vi "Graph_Peak_testing.vi"(6 "CSV file path":path, 7 "error in":errorcluster, 10 "Cluster":T2) -> (0 "MIN_MAX_BPM":bool, 2 "Filter Graph":cluster{timestamp[], ext[]}(graph), 3 "MIN_MAX_PRESSURE":bool, 4 "ACTUAL BPM":dbl, 5 "error out":errorcluster, 8 "MAX_MIN_PRESSURE":cluster{"MIN":dbl, "MAX":dbl, "ACTUAL":dbl}, 9 "UnFiltered \nSize":i32)   [LabVIEW 2017]
uses:
  <vilib>/Utility/file.llb/Read Delimited Spreadsheet (string).vi
panel:
  out "Pressure":T1
  out "ACTUAL":ext
  out "max value 2":ext
  out "max value":ext
  out "Peak samples / second":dbl
  out "time in sec between start peak stop peak":dbl
  out "Array 14":ext[](array[numeric])
  out "Array":timestamp[](array[timestamp])
  out "input filter array":ext[](array[numeric])
  out "Normal Graph":cluster{timestamp[], ext[]}(graph)
  out "Numeric 3":i32
  out "Numeric":i32
  out "Array 13":ext[][](array[numeric])
  out "Array 12":ext[](array[numeric])
  out "appended array 2":timestamp[][](array[timestamp])
  out "peak count":i32
  out "Array 11":ext[](array[numeric])
  out "Array 8":timestamp[](array[timestamp])
  out "appended array":timestamp[][](array[timestamp])
  out "Array 9":ext[][](array[numeric])
  out "Input\nLower\nthan\nthreshold":bool
  out "Filtered \nSize":i32
  out "STOP\nTHRESHOLD\nTRIGGER\nindex":i32
  out "START\nTHRESHOLD\nTRIGGER\nindex":i32
  out "time stamp":timestamp[](array[timestamp])
  out "input unfilter array":ext[](array[numeric])
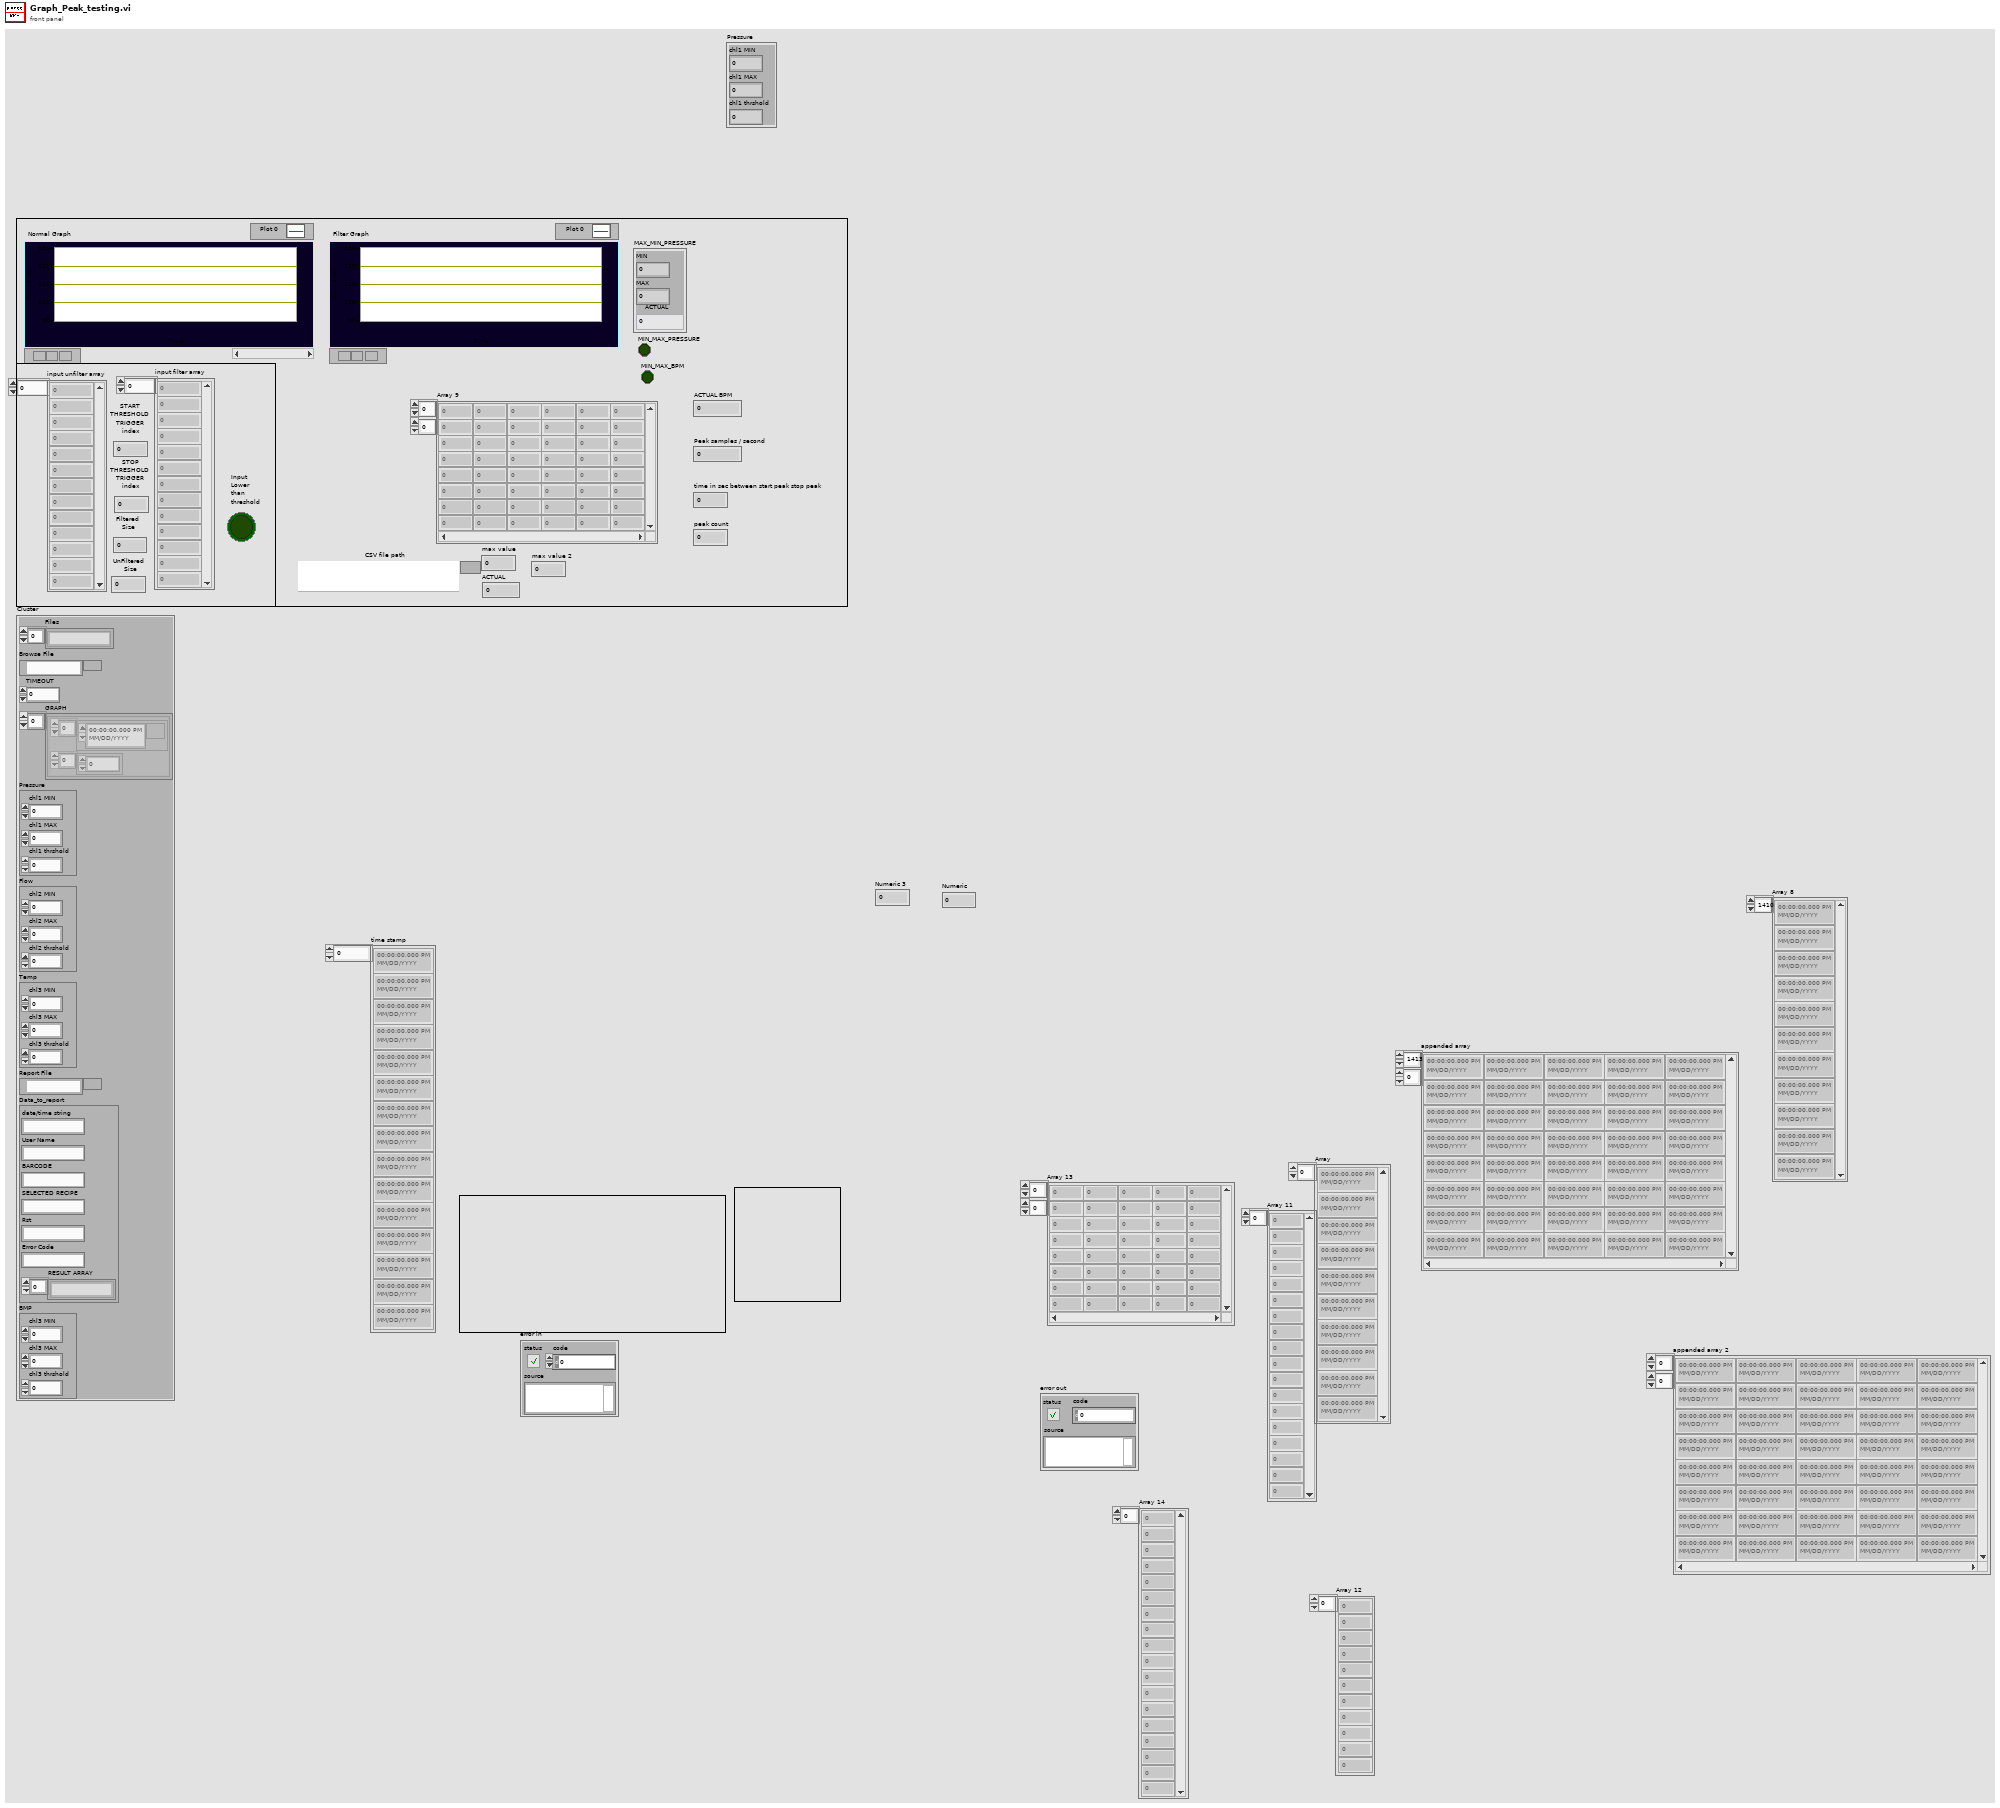
[diagram p1: front panel]
types:
  T1 = cluster{"chl1 MIN":dbl, "chl1 MAX":dbl, "chl1 thrshold":dbl}
  T2 = cluster{"Files":string[], "Browse File":path, "TIMEOUT":i32, "GRAPH":cluster{timestamp[], ext[]}[], "Pressure":cluster{"chl1 MIN":dbl, "chl1 MAX":dbl, "chl1 thrshold":dbl}, "Flow":cluster{"chl2 MIN":dbl, "chl2 MAX":dbl, "chl2 thrshold":dbl}, "Temp":cluster{"chl3 MIN":dbl, "chl3 MAX":dbl, "chl3 thrshold":dbl}, "Report File":path, "Data_to_report":cluster{"date/time string":string, "User Name":string, "BARCODE":string, "SELECTED RECIPE":string, "Rst":string, "Error Code":string, "RESULT ARRAY":string[]}, "BMP":cluster{"chl3 MIN":dbl, "chl3 MAX":dbl, "chl3 thrshold":dbl}}
  T3 = cluster{"chl3 MIN":dbl, "chl3 MAX":dbl, "chl3 thrshold":dbl}
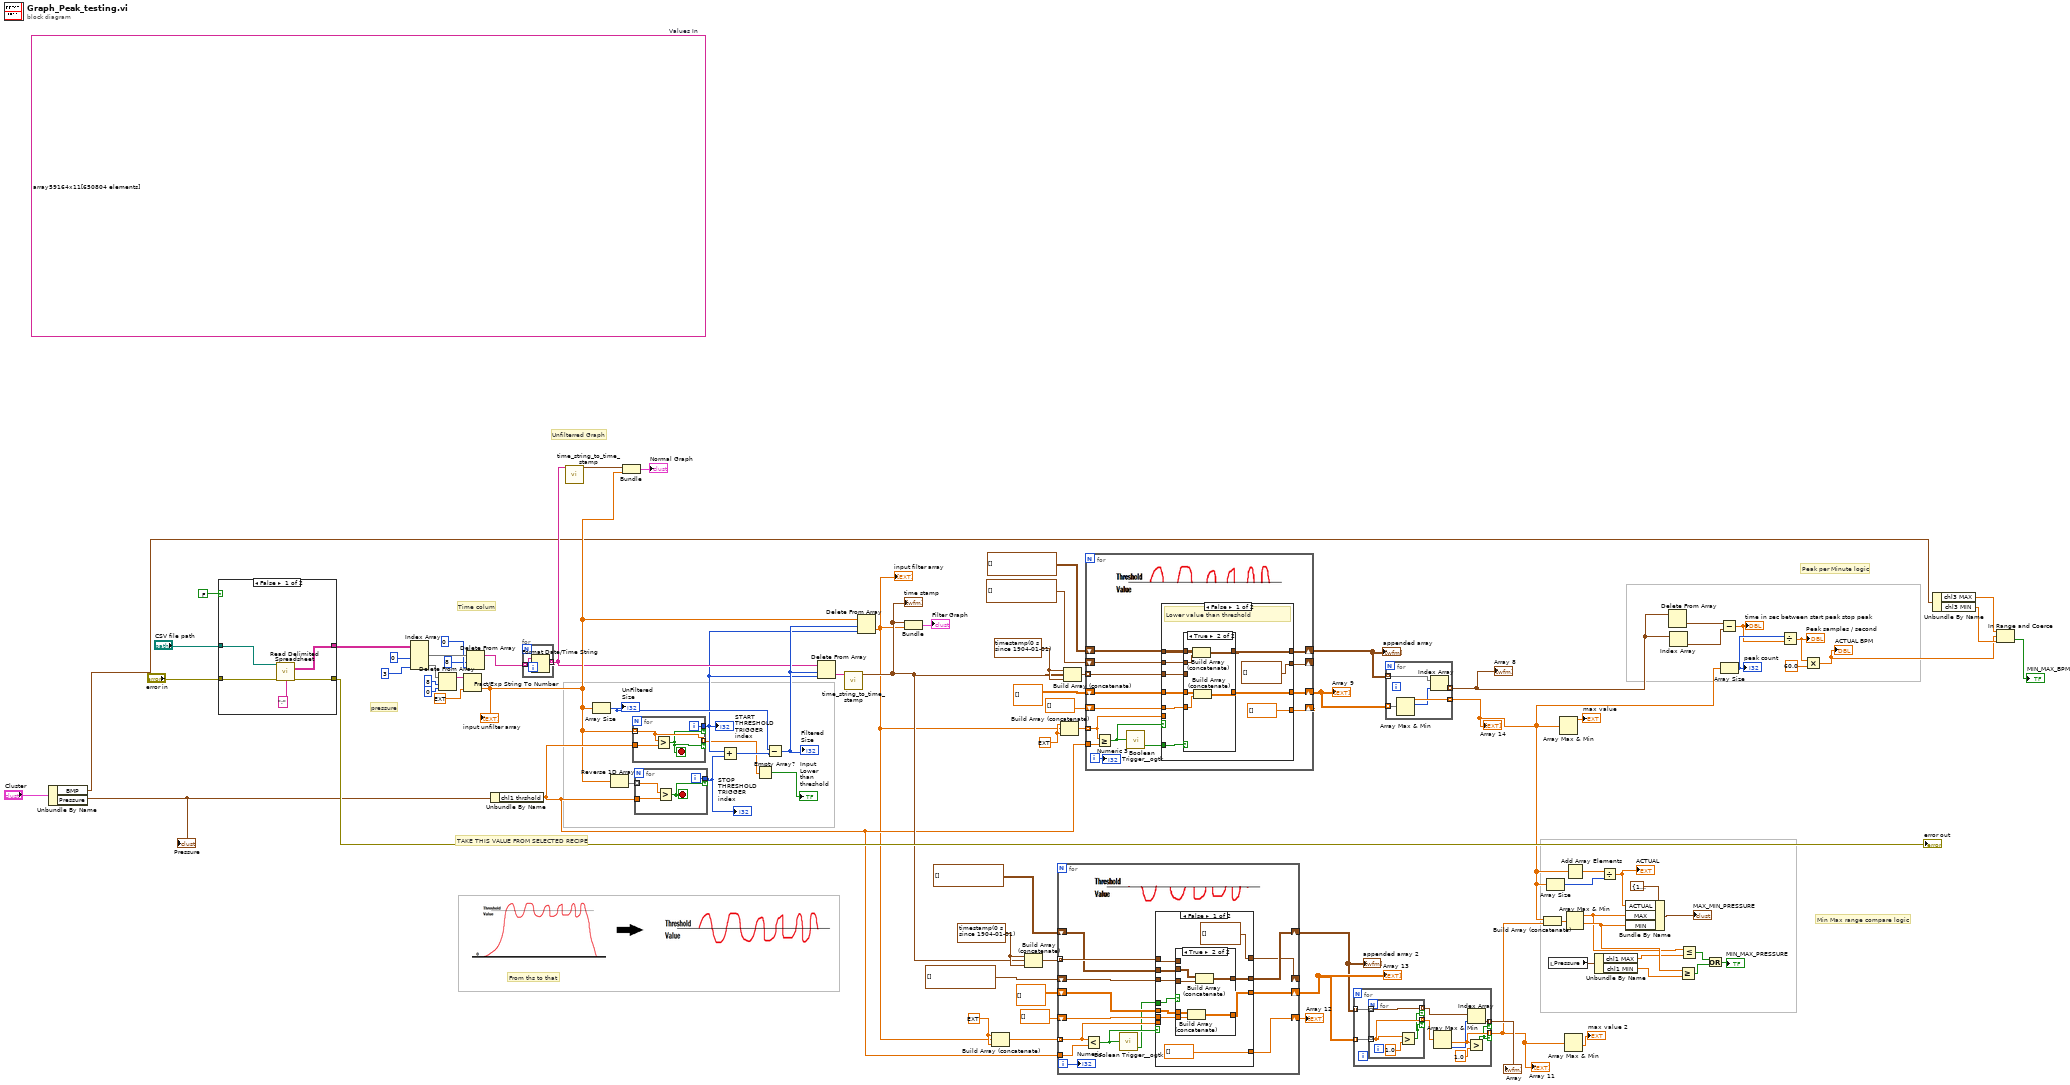
[diagram p0: block diagram]
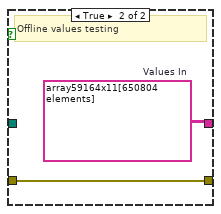
[diagram p2: hidden frame]
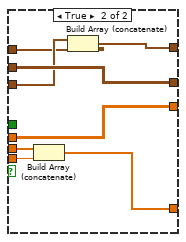
[diagram p4: hidden frame]
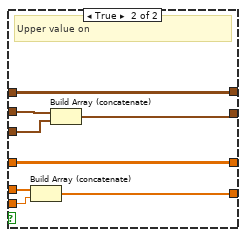
[diagram p6: hidden frame]
diagram:
  (unwired) string[][] array59164x11[650804 elements]  # Values In
  w62 = timestamp(0 s since 1904-01-01) ("time stamp")
  w61 = ext 0.0 ("String")
  w69 = timestamp(0 s since 1904-01-01) ("time stamp")
  w70 = ext 0.0 ("String")
  # "Min Max range compare logic"
  # "Peak per Minute logic"
  # "Unfilterred Graph"
  # "From ths to that"
  # "pressure"
  # "Time colum"
  # "TAKE THIS VALUE FROM SELECTED RECIPE"
  n1 = Unbundle By Name("Cluster") -> ("BMP"=w5:T3, "Pressure"=w6:T1)
  "Pressure" <- w6
  n2 = case shown="False" FALSE {
    tunnel: [w91 w94] -> w82
    tunnel: "CSV file path" -> [w90 _]
    tunnel: [w89 w93] -> w52
    tunnel: "error in" -> [w88 w93]
    frame False {
      n3 = call-poly <vilib>:"Read Delimited Spreadsheet.vi"("file path (dialog if empty)"=w90, "error in (no error)"=w88, "delimiter (\\t)"=";" ("delimiter (\\t)")) -> ("all rows"=w91:string[][], "error out"=w89:errorcluster)  [unwired: 7 in, 4 out]
    }
    frame True {
      w94 = string[][] array59164x11[650804 elements]  # Values In
      # "Offline values testing"
    }
  }
  "error out" <- w52
  n4 = Index Array(array=w82, index (col) #1=0 ("index (row)"), index (col) #2=3 ("index (row)")) -> (element #1=w87:string[], element #2=w83:string[])  [unwired: 2 in]
  n5 = Delete From Array(array=w83, length=8 ("index (row)"), index=0 ("index (row)")) -> (array with subset deleted=w78:string[])  [unwired: 1 out]
  n6 = Fract/Exp String To Number(string=w78, default (0 dbl)=ext 0.0 ("String")) -> (number=w43:ext[])  [unwired: 2 in, 1 out]
  "input unfilter array" <- w43
  n7 = Delete From Array(array=w87, length=8 ("index (row)"), index=0 ("index (row)")) -> (array with subset deleted=w41:string[])  [unwired: 1 out]
  n8 = Unbundle By Name(w6) -> ("chl1 thrshold"=w48:dbl)
  n9 = for {
    tunnel: w41 -> [w96] mode=indexing
    tunnel: [w95] -> w38 mode=indexing
    n10 = Format Date/Time String(time format string (%c)=w96) -> (date/time string=w95:string)  [unwired: 2 in]
  }
  n11 = call "time_string_to_time_stamp.vi"("Array in"=w38) -> ("Array out"=w39:timestamp[])  [unwired: 10 in]
  n12 = Array Size(array=w43) -> (size(s)=w40:i32)
  "UnFiltered \nSize" <- w40
  n13 = Reverse 1D Array(array=w43) -> (reversed array=w77:ext[])
  n14 = Bundle("Array out"=w39, w43) -> (→"Normal Graph":cluster{"Array out":timestamp[], ext[]})  [unwired: 1 in]
  n15 = for {
    tunnel: w43 -> [w98] mode=indexing
    tunnel: [w100] -> w25 if=w97
    tunnel: w48 -> [w99]
    tunnel: [w98] -> w23 mode=indexing if=w97
    i -> [w100]
    stop <- w97 stop-if-true
    n16 = Greater?(x=w98, y=w99) -> (0:w97:bool)
  }
  "START\nTHRESHOLD\nTRIGGER\nindex" <- w25
  n17 = for {
    tunnel: w77 -> [w104] mode=indexing
    tunnel: [w103] -> w76 if=w102
    tunnel: w48 -> [w101]
    i -> [w103]
    stop <- w102 stop-if-true
    n18 = Greater?(x=w104, y=w101) -> (0:w102:bool)
  }
  "STOP\nTHRESHOLD\nTRIGGER\nindex" <- w76
  n19 = Add(x=w25, y=w76) -> (x+y=w75:i32)
  n20 = Empty Array?(array=w23) -> (empty?=→"Input\nLower\nthan\nthreshold":bool)
  n21 = Subtract(x=w40, y=w75) -> (x-y=w74:i32)
  "Filtered \nSize" <- w74
  n22 = Delete From Array(array=w38, length=w74, index=w25) -> (deleted portion=w49:string[])  [unwired: 1 out]
  n23 = call "time_string_to_time_stamp.vi"("Array in"=w49) -> ("Array out"=w50:timestamp[])  [unwired: 10 in]
  "time stamp" <- w50
  n24 = Delete From Array(array=w43, length=w74, index=w25) -> (deleted portion=w42:ext[])  [unwired: 1 out]
  "input filter array" <- w42
  n25 = Bundle("Array out"=w50, w42) -> (→"Filter Graph":cluster{"Array out":timestamp[], ext[]})  [unwired: 1 in]
  n26 = Build Array (concatenate)(w61, w42, w61) -> (w60:ext[])
  n27 = Build Array (concatenate)(w62, w50, w62) -> (w65:timestamp[])
  n28 = for {
    tunnel: w60 -> [w116] mode=indexing
    tunnel: w48 -> [w118]
    shift-right: [w115] -> w59
    shift-left: ext[] [] -> [w114]
    shift-right: [w112] -> w56
    shift-left: ext[][] [] -> [w113]
    tunnel: w65 -> [w110] mode=indexing
    shift-right: [w109] -> w55
    shift-left: timestamp[][] [] ("appended array") -> [w108]
    shift-right: [w106] -> _
    shift-left: timestamp[] [] ("appended array") -> [w107]
    i -> [w105]
    n29 = Less?(x=w116, y=w118) -> (x < y?=w117:bool)
    n30 = call <userlib>:"Boolean Trigger__ogtk.vi"("Boolean Input"=w117) -> ("Falling Edge"=w111:bool)  [unwired: 1 in, 1 out]
    n31 = case shown="False" w117 {
      tunnel: w116 -> [_ w144]
      tunnel: [ext[] [] w143] -> w115
      tunnel: w114 -> [w125 w141]
      tunnel: w113 -> [w126 w142]
      tunnel: [w127 w142] -> w112
      tunnel: w111 -> [w124 _]
      tunnel: w110 -> [w123 w137]
      tunnel: [w122 w140] -> w109
      tunnel: w108 -> [w121 w140]
      tunnel: w107 -> [w120 w138]
      tunnel: [timestamp[] [] ("appended array") w139] -> w106
      frame False {
        n32 = case shown="True" w124 {
          tunnel: [w130 w136] -> w127
          tunnel: w126 -> [w130 w135]
          tunnel: w125 -> [_ w134]
          tunnel: w123 -> [_ _]
          tunnel: [w129 w133] -> w122
          tunnel: w121 -> [w129 w132]
          tunnel: w120 -> [_ w131]
          frame False {
          }
          frame True {
            n33 = Build Array (concatenate)(w135, w134) -> (w136:ext[][])
            n34 = Build Array (concatenate)(w132, w131) -> (w133:timestamp[][])
          }
        }
      }
      frame True {
        n35 = Build Array (concatenate)(w141, w144) -> (w143:ext[])
        n36 = Build Array (concatenate)(w138, w137) -> (w139:timestamp[])
      }
    }
    "Numeric" <- w105
  }
  "Array 13" <- w56
  "Array 12" <- w59
  "appended array 2" <- w55
  n37 = Build Array (concatenate)(w70, w42, w70) -> (w71:ext[])
  n38 = Build Array (concatenate)(w69, w50, w69) -> (w66:timestamp[])
  n39 = for {
    tunnel: w71 -> [w156] mode=indexing
    tunnel: w48 -> [w158]
    shift-right: [w145] -> _
    shift-left: ext[] [] -> [w155]
    shift-right: [w147] -> w36
    shift-left: ext[][] [] -> [w154]
    tunnel: w66 -> [w152] mode=indexing
    shift-right: [w148] -> w37
    shift-left: timestamp[][] [] ("appended array") -> [w151]
    shift-right: [w146] -> _
    shift-left: timestamp[] [] ("appended array") -> [w150]
    i -> [w149]
    n40 = Greater Or Equal?(x=w156, y=w158) -> (x >= y?=w157:bool)
    n41 = call <userlib>:"Boolean Trigger__ogtk.vi"("Boolean Input"=w157) -> ("Falling Edge"=w153:bool)  [unwired: 1 in, 1 out]
    n42 = case shown="False" w157 {
      tunnel: w156 -> [_ w184]
      tunnel: [ext[] [] w183] -> w145
      tunnel: w155 -> [w165 w181]
      tunnel: w154 -> [w166 w182]
      tunnel: [w167 w182] -> w147
      tunnel: w153 -> [w164 _]
      tunnel: w152 -> [w163 w177]
      tunnel: [w162 w180] -> w148
      tunnel: w151 -> [w161 w180]
      tunnel: w150 -> [w160 w178]
      tunnel: [timestamp[] [] ("appended array") w179] -> w146
      frame False {
        # "Lower value than threshold"
        n43 = case shown="True" w164 {
          tunnel: [w170 w176] -> w167
          tunnel: w166 -> [w170 w175]
          tunnel: w165 -> [_ w174]
          tunnel: w163 -> [_ _]
          tunnel: [w169 w173] -> w162
          tunnel: w161 -> [w169 w172]
          tunnel: w160 -> [_ w171]
          frame False {
          }
          frame True {
            n44 = Build Array (concatenate)(w172, w171) -> (w173:timestamp[][])
            n45 = Build Array (concatenate)(w175, w174) -> (w176:ext[][])
          }
        }
      }
      frame True {
        # "Upper value on"
        n46 = Build Array (concatenate)(w181, w184) -> (w183:ext[])
        n47 = Build Array (concatenate)(w178, w177) -> (w179:timestamp[])
      }
    }
    "Numeric 3" <- w149
  }
  "Array 9" <- w36
  "appended array" <- w37
  n48 = for {
    tunnel: w56 -> [w190] mode=indexing
    tunnel: w55 -> [w192] mode=indexing
    tunnel: [w186] -> w21 mode=indexing if=w185
    tunnel: [w193] -> w35 mode=indexing if=w185
    n49 = for {
      tunnel: w190 -> [w195] mode=indexing
      tunnel: [w196] -> w191 mode=indexing if=w194
      tunnel: w192 -> [w196] mode=indexing
      tunnel: [w195] -> w189 mode=indexing if=w194
      n50 = Greater?(x=w195, y=1.0) -> (0:w194:bool)
    }
    n51 = Array Max & Min(array=w189) -> (min value=w186:ext, min index (indices)=w187:i32)  [unwired: 2 out]
    n52 = Index Array(array=w191, index=w187) -> (element=w193:timestamp)
    n53 = Greater?(x=w186, y=1.0) -> (0:w185:bool)
  }
  "Array 11" <- w21
  "Array" <- w35
  n54 = for {
    tunnel: w36 -> [w202] mode=indexing
    tunnel: w37 -> [w200] mode=indexing
    tunnel: [w201] -> w11 mode=indexing
    tunnel: [w198] -> w32 mode=indexing
    n55 = Array Max & Min(array=w202) -> (max value=w201:ext, max index (indices)=w199:i32)  [unwired: 2 out]
    n56 = Index Array(array=w200, index=w199) -> (element=w198:timestamp)
  }
  "Array 8" <- w32
  "Array 14" <- w11
  n57 = Build Array (concatenate)(w11, w21) -> (w34:ext[])
  n58 = Array Size(array=w11) -> (size(s)=w8:i32)
  n59 = local read "Pressure"() -> (w3:T1)
  n60 = Array Max & Min(array=w11) -> (max value=→"max value":ext)  [unwired: 3 out]
  n61 = Array Max & Min(array=w21) -> (min value=→"max value 2":ext)  [unwired: 3 out]
  n62 = Array Max & Min(array=w34) -> (max value=w13:ext, min value=w14:ext)  [unwired: 2 out]
  n63 = Add Array Elements(numeric array=w11) -> (sum=w9:ext)
  n64 = Unbundle By Name(w3) -> ("chl1 MAX"=w2:dbl, "chl1 MIN"=w1:dbl)
  n65 = Divide(x=w9, y=w8) -> (x/y=w10:ext)
  "ACTUAL" <- w10
  n66 = Bundle By Name(cluster=cluster{"MIN":dbl, "MAX":dbl, "ACTUAL":dbl} {"MIN"=110.0, "MAX"=130.0, "ACTUAL"=0.0} ("CHL 2"), "ACTUAL"=w10, "MAX"=w13, "MIN"=w14) -> (→"MAX_MIN_PRESSURE":cluster{"MIN":dbl, "MAX":dbl, "ACTUAL":dbl})
  n67 = Delete From Array(array=w32) -> (deleted portion=w31:timestamp)  [unwired: 2 in, 1 out]
  n68 = Index Array(array=w32) -> (element=w30:timestamp)  [unwired: 1 in]
  n69 = Greater Or Equal?(x=w14, y=w1) -> (x >= y?=w15:bool)
  n70 = Less Or Equal?(x=w13, y=w2) -> (x <= y?=w12:bool)
  n71 = Or(x=w12, y=w15) -> (x .or. y?=→"MIN_MAX_PRESSURE":bool)
  n72 = Subtract(x=w31, y=w30) -> (x-y=w28:dbl)
  "time in sec between start peak stop peak" <- w28
  n73 = Array Size(array=w11) -> (size(s)=w29:i32)
  "peak count" <- w29
  n74 = Divide(x=w29, y=w28) -> (x/y=w27:dbl)
  "Peak samples / second" <- w27
  n75 = Multiply(x=w27, y=60.0) -> (x*y=w17:dbl)
  "ACTUAL BPM" <- w17
  n76 = Unbundle By Name(w5) -> ("chl3 MAX"=w19:dbl, "chl3 MIN"=w18:dbl)
  n77 = In Range and Coerce(upper limit=w19, x=w17, lower limit=w18) -> (In Range?=→"MIN_MAX_BPM":bool)  [unwired: 1 out]
